vi "Write mods.vi"(8 "error in":errorcluster, 10 "mods":refnum<class "VI modification.lvclass">[](array[class]), 11 "modification container in":refnum<class "modification container.lvclass">) -> (0 "error out":errorcluster, 3 "modification container out":refnum<class "modification container.lvclass">)   [LabVIEW 2013, in "modification container.lvclass"]
uses:
  modification container.lvclass
  VI modification.lvclass
  modification container.lvclass/modification container.ctl
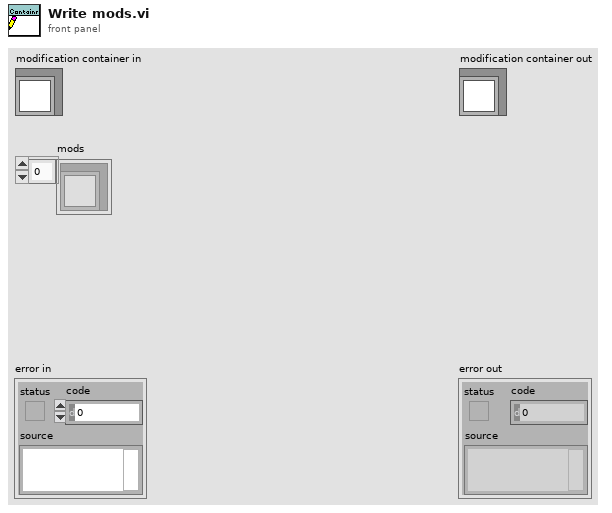
[diagram p1: front panel]
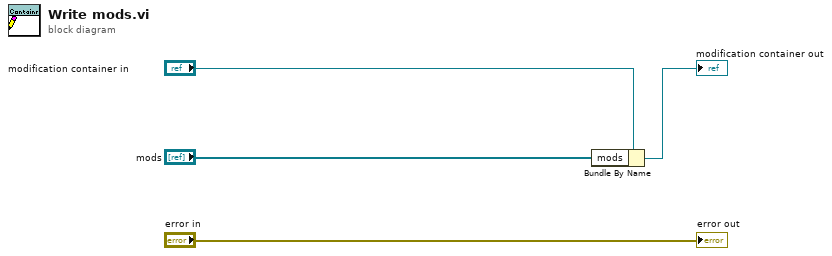
[diagram p0: block diagram]
diagram:
  n1 = Bundle By Name(cluster="modification container in", "mods"="mods") -> (→"modification container out":refnum<class "modification container.lvclass">)
  "error out" <- "error in"
